vi "SVT Running Leq Sound Level.vi"   [LabVIEW 2017]
doc: "Computes the running equivalent continuous sound level (Leq) of <B>scaled signal [EU]</B>. A new running Leq value is returned each time you call this VI. You can use this polymorphic VI to compute the running Leq for a single channel or for N channels. The data type you wire to the <B>scaled signal [EU]</B> input determines the polymorphic instance to use."
uses:
  <vilib>/addons/Sound and Vibration/svt_Level/SoundVib_SoundLevel.lvlib
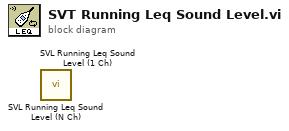
[diagram p0: block diagram]
diagram:
  n1 = call <vilib>:"SVL Running Leq Sound Level (N Ch).vi"() -> ()  [unwired: 8 in, 4 out]
  n2 = call <vilib>:"SVL Running Leq Sound Level (1 Ch).vi"() -> ()  [unwired: 8 in, 4 out]
